vi "Helper Main.vi"(11 "Events":T1) -> ()   [LabVIEW 2020, in "Test.Maui 2.0.Panels.lvclass"]
uses:
  Test.Maui 2.0.Panels/Test.Maui 2.0.Panels.lvclass
panel:
  in  "Ring 2":u16(ring)
  in  "Ring":u16(ring)
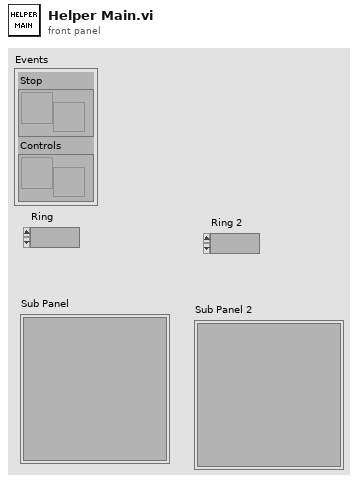
[diagram p1: front panel]
types:
  T1 = cluster{"Stop":refnum<user-event>, "Controls":refnum<user-event>}
  T2 = cluster{"Ring":refnum<vi>, "Sub Panel":refnum<vi>}
  T3 = cluster{"Ring 2":refnum<vi>, "Sub Panel 2":refnum<vi>}
  T4 = cluster{"Ring 2":refnum<vi>, "Sub Panel 2":refnum<vi>}[]
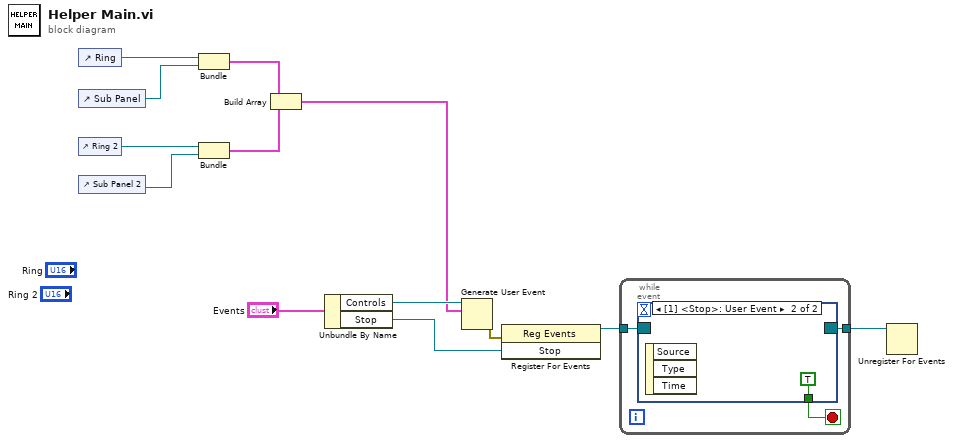
[diagram p0: block diagram]
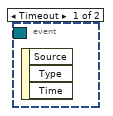
[diagram p2: hidden frame]
diagram:
  n1 = control-ref of="Ring"() -> (w11:refnum<vi>)
  n2 = control-ref of="Sub Panel"() -> (w10:refnum<vi>)
  n3 = control-ref of="Ring 2"() -> (w13:refnum<vi>)
  n4 = control-ref of="Sub Panel 2"() -> (w12:refnum<vi>)
  n5 = Bundle("Ring"=w11, "Sub Panel"=w10) -> (w9:T2)  [unwired: 1 in]
  n6 = Bundle("Ring 2"=w13, "Sub Panel 2"=w12) -> (w8:T3)  [unwired: 1 in]
  n7 = Build Array(w9, w8) -> (w1:T4)
  n8 = Unbundle By Name("Events") -> ("Controls"=w4:refnum<user-event>, "Stop"=w5:refnum<user-event>)
  n9 = Generate User Event(user event=w4, event data cluster=w1) -> (error out=w3:errorcluster)  [unwired: 2 in, 1 out]
  n10 = register-events(error in=w3, w5) -> (reference out=w7:refnum<event-registration>)  [unwired: 1 in, 1 out]
  n11 = while {
    tunnel: w7 -> [w16]
    tunnel: [w14] -> w2
    stop <- w15 stop-if-true
    n12 = event shown="[1] <Stop>: User Event" {
      selector: w16 -> [_ _]
      dyn-events: [_ _] -> w14
      timeout: _ -> [_ _]
      tunnel: [_ TRUE] -> w15
      event Timeout {
        n13 = event-data() -> ()  [unwired: 1 in, 3 out]
      }
      event User Event {
        n14 = event-data() -> ()  [unwired: 1 in, 3 out]
      }
    }
  }
  n15 = Unregister For Events(event registration refnum=w2) -> ()  [unwired: 1 in, 1 out]
